vi "Unicode String Probe (Extended).vi"(11 "String":string) -> (2 "Value String":string, 3 "Boolean":bool)   [LabVIEW 2020]
uses:
  Unicode/Controls/String Encoding.ctl
  Private/Conversion/Text to UTF-8.vi
  Private/Conversion/Polymorphic VIs/Text to UTF-8 (LabVIEW String).vi
  Private/Conversion/Encoded UTF-8 String to Encoded UTF-16LE String.vi
  Unicode/SubVIs/UTF-16 Byte Swap.vi
  Private/Conversion/UTF-8 to Text.vi
  Private/Conversion/Polymorphic VIs/UTF-8 to Text (LabVIEW String).vi
  Private/Conversion/Encoded UTF-16LE String to Encoded UTF-8 String.vi
  Unicode/SubVIs/Byte Order Marks.vi
  Unicode/Strip BOM.vi
  Unicode/Detect String Encoding.vi/f4e2713d-ca87-487a-b901-d606fc3002c3.vi
  Private/Library/gu_is_text_utf16.vi
  Private/Library/gu_is_text_utf8.vi
  G-Unicode.lvlib
panel:
  out "Input Length":i32
  out "Truncated":bool
  out "ANSI":string
  out "UTF-16BE":string
  out "UTF-16LE":string
  out "UTF-8":string
  out "Byte Order Mark":bool
  out "Detected Encoding":T1=enum."Unknown"
  out "Raw Bytes":u8[](array[numeric]) format="%02x"
  out "Raw String":string
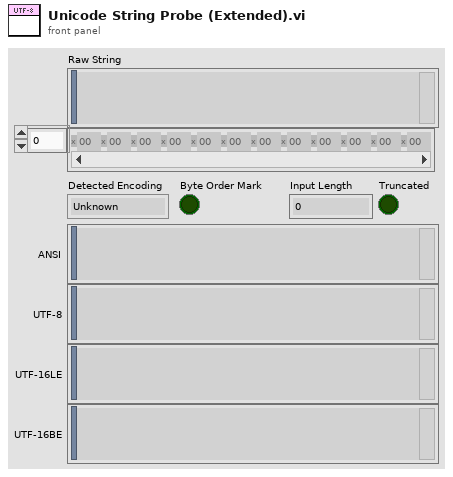
[diagram p1: front panel]
types:
  T1 = typedef "G-Unicode.lvlib/String Encoding.ctl" = enum16{"ANSI", "UTF-8", "UTF-16LE", "UTF-16BE", "Unknown"}
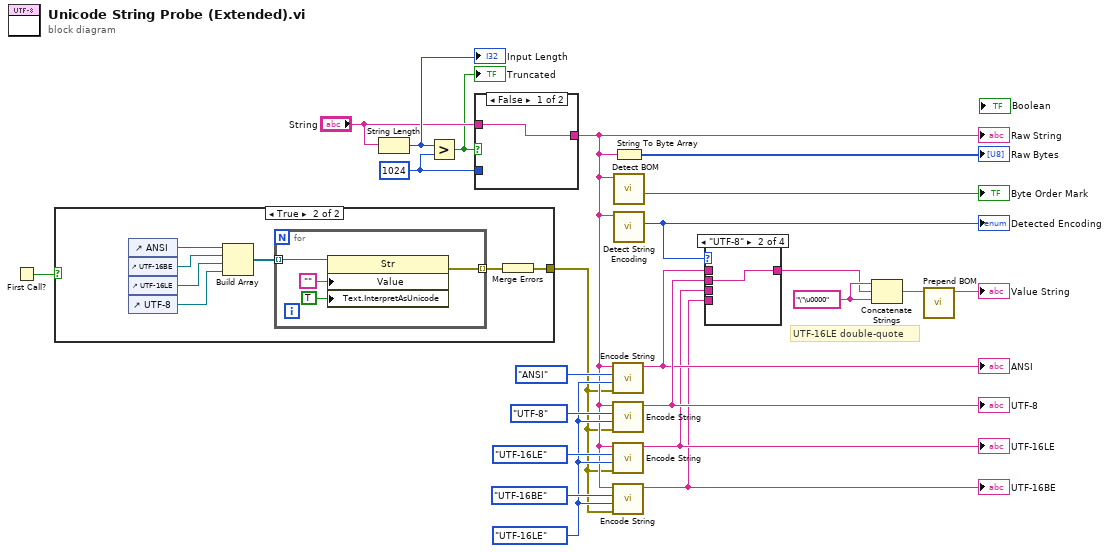
[diagram p0: block diagram]
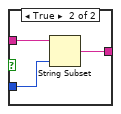
[diagram p3: hidden frame]
diagram:
  w4 = "\"\u0000" ("string")
  w9 = 1024 ("y")
  w14 = String_Encoding."UTF-16LE" ("Output Encoding (UTF-8)")
  # "UTF-16LE double-quote"
  n1 = First Call?() -> (First Call?: T/F=w1:bool)
  n2 = case shown="True" w1 {
    tunnel: [_ w30] -> w6
    frame False {
    }
    frame True {
      n3 = control-ref of="ANSI"() -> (w29:refnum<vi>)
      n4 = control-ref of="UTF-16BE"() -> (w28:refnum<vi>)
      n5 = control-ref of="UTF-16LE"() -> (w27:refnum<vi>)
      n6 = control-ref of="UTF-8"() -> (w26:refnum<vi>)
      n7 = Build Array(w29, w28, w27, w26) -> (w25:refnum<vi>[])
      n8 = for {
        tunnel: w25 -> [w31] mode=indexing
        tunnel: [w34] -> w24 mode=indexing
        n9 = property on="Property Node" class="Str"(reference=w31, "Value"="", "Text.InterpretAsUnicode"=TRUE ("Text.Interpret As Unicode")) -> (error out=w34:errorcluster)  [unwired: 1 in, 1 out]
      }
      n10 = Merge Errors(w24) -> (w30:errorcluster)
    }
  }
  n11 = String Length(string="String") -> (length=w10:i32)
  "Input Length" <- w10
  n12 = Greater?(x=w10, y=w9) -> (0:w5:bool)
  "Truncated" <- w5
  n13 = case shown="False" w5 {
    tunnel: "String" -> [w35 w38]
    tunnel: w9 -> [_ w37]
    tunnel: [w35 w36] -> w8
    frame False {
    }
    frame True {
      n14 = String Subset(string=w38, length (rest)=w37) -> (substring=w36:string)  [unwired: 1 in]
    }
  }
  "Raw String" <- w8
  n15 = call "Encode String.vi"("error in"=w6, "Output Encoding (UTF-16LE)"=w14, "Input Encoding (ANSI)"=String_Encoding."ANSI", "String in"=w8) -> ("String out"=w13:string)  [unwired: 6 in, 1 out]
  "ANSI" <- w13
  n16 = call "Encode String.vi"("error in"=w6, "Output Encoding (UTF-16LE)"=w14, "Input Encoding (ANSI)"=String_Encoding."UTF-8", "String in"=w8) -> ("String out"=w16:string)  [unwired: 6 in, 1 out]
  "UTF-8" <- w16
  n17 = call "Encode String.vi"("error in"=w6, "Output Encoding (UTF-16LE)"=w14, "Input Encoding (ANSI)"=String_Encoding."UTF-16LE", "String in"=w8) -> ("String out"=w12:string)  [unwired: 6 in, 1 out]
  "UTF-16LE" <- w12
  n18 = call "Encode String.vi"("error in"=w6, "Output Encoding (UTF-16LE)"=w14, "Input Encoding (ANSI)"=String_Encoding."UTF-16BE", "String in"=w8) -> ("String out"=w11:string)  [unwired: 6 in, 1 out]
  "UTF-16BE" <- w11
  n19 = String To Byte Array(string=w8) -> (unsigned byte array=→"Raw Bytes":u8[])
  n20 = call "Detect BOM.vi"("String"=w8) -> ("BOM Found"=→"Byte Order Mark":bool)  [unwired: 9 in, 1 out]
  n21 = call "Detect String Encoding.vi"("String"=w8) -> ("Encoding"=w19:T1)  [unwired: 8 in, 2 out]
  "Detected Encoding" <- w19
  n22 = case shown="\"UTF-8\"" w19 {
    tunnel: w16 -> [_ w40 _ _]
    tunnel: [w39 w40 w41 w42] -> w2
    tunnel: w12 -> [_ _ w41 _]
    tunnel: w11 -> [_ _ _ w42]
    tunnel: w13 -> [w39 _ _ _]
    frame "ANSI", Default {
    }
    frame "UTF-8" {
    }
    frame "UTF-16LE" {
    }
    frame "UTF-16BE" {
    }
  }
  n23 = Concatenate Strings(w4, w2, w4) -> (w3:string)
  n24 = call "Prepend BOM.vi"("String"=w3) -> ("String with BOM"=→"Value String":string)  [unwired: 9 in, 1 out]
